vi "Get all Library Public VI Names.vi"(8 "error in (no error)":errorcluster, 11 "Library or Class Path":path) -> (0 "error out":errorcluster, 3 "Public VI Names":string[](array[string]))   [LabVIEW 2020, in "TEST JKI State Machine API.lvlib"]
uses:
  TEST JKI State Machine API.lvlib
  <userlib>/_OpenG.lib/file/file.llb/Strip Path Extension - String__ogtk.vi
  <userlib>/_OpenG.lib/file/file.llb/openg_file.lvlib
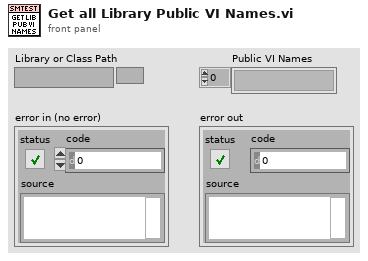
[diagram p1: front panel]
types:
  T1 = enum32{"invalid scope", "public", "private", "protected", "community"}
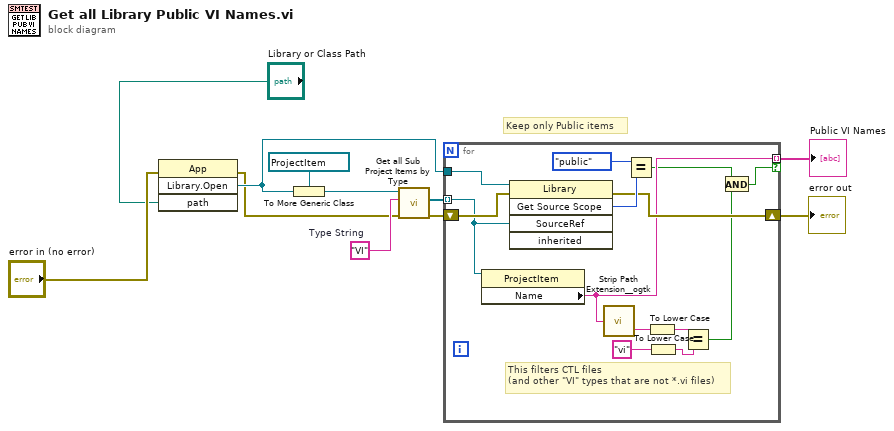
[diagram p0: block diagram]
diagram:
  w5 = "VI"  # Type String
  # "Keep only Public items"
  n1 = invoke class="App" method="Library.Open"(error in="error in (no error)", "path"="Library or Class Path") -> (error out=w4:errorcluster, "Open Library"=w7:refnum<vi>)  [unwired: 2 in, 2 out]
  n2 = To More Generic Class(target class=refnum<vi> refnum ("reference"), reference=w7) -> (generic class reference=w3:refnum<vi>)
  n3 = call "Get all Sub Project Items by Type.vi"("error in (no error)"=w4, "Type String"=w5, "ProjectItem"=w3) -> ("error out"=w8:errorcluster, "Project Items"=w6:refnum<vi>[])  [unwired: 7 in]
  n4 = for {
    tunnel: w6 -> [w20] mode=indexing
    tunnel: w7 -> [w25]
    shift-right: [w21] -> w10
    shift-left: w8 -> [w24]
    tunnel: [w19] -> w9 mode=indexing if=w12
    # "This filters CTL files\n(and other \"VI\" types that are not *.vi files)"
    n5 = property class="ProjectItem"(reference=w20) -> ("Name"=w19:string)  [unwired: 1 in, 2 out]
    n6 = invoke class="Library" method="Get Source Scope"(reference=w25, error in=w24, "SourceRef"=w20) -> (error out=w21:errorcluster, "GetSourceScope"=w23:T1)  [unwired: 2 in, 3 out]
    n7 = call-poly <userlib>:"Strip Path Extension__ogtk.vi"("path"=w19) -> ("extension"=w18:string)  [unwired: 1 out]
    n8 = Equal?(x=T1."public" ("Source Scope:Get"), y=w23) -> (x = y?=w13:bool)
    n9 = To Lower Case(string=w18) -> (all lower case string=w15:string)
    n10 = To Lower Case(string="vi") -> (all lower case string=w16:string)
    n11 = Equal?(x=w15, y=w16) -> (x = y?=w14:bool)
    n12 = And(x=w13, y=w14) -> (x .and. y?=w12:bool)
  }
  "error out" <- w10
  "Public VI Names" <- w9
